vi "Format VI Information.vi"(0 "string in":string, 1 "output dir":path, 5 "file paths":path[](array[path]), 7 "image dir":path, 11 "error in":errorcluster) -> (4 "string out":string, 15 "error out":errorcluster)   [LabVIEW 2019, in "MD Generator.lvlib"]
uses:
  MD Generator.lvlib
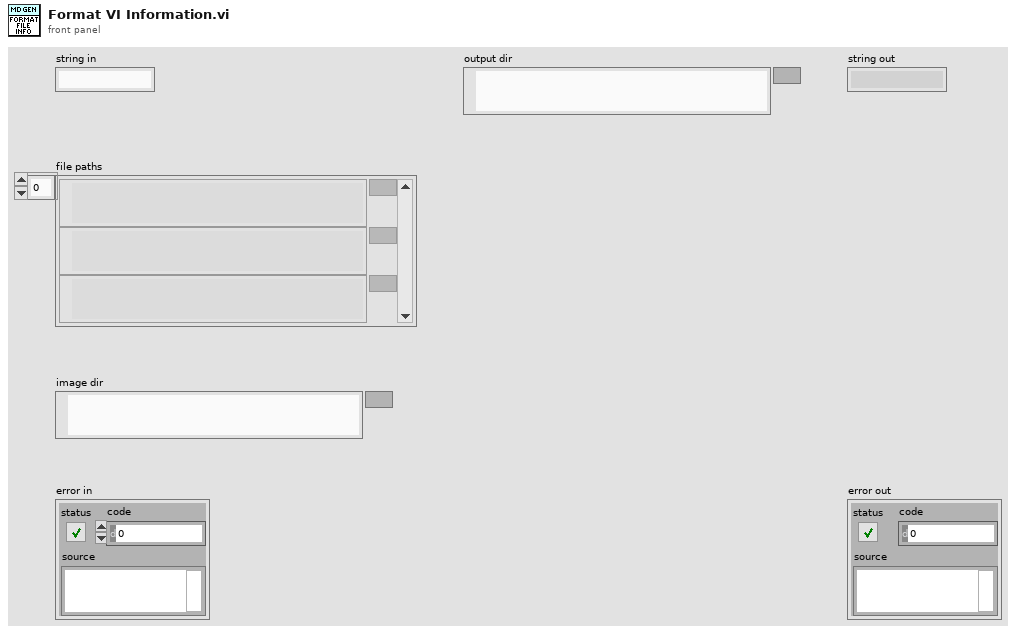
[diagram p1: front panel]
types:
  T1 = enum32{"Custom", "Standard", "Using Panel", "Using SubVI", "Complete"}
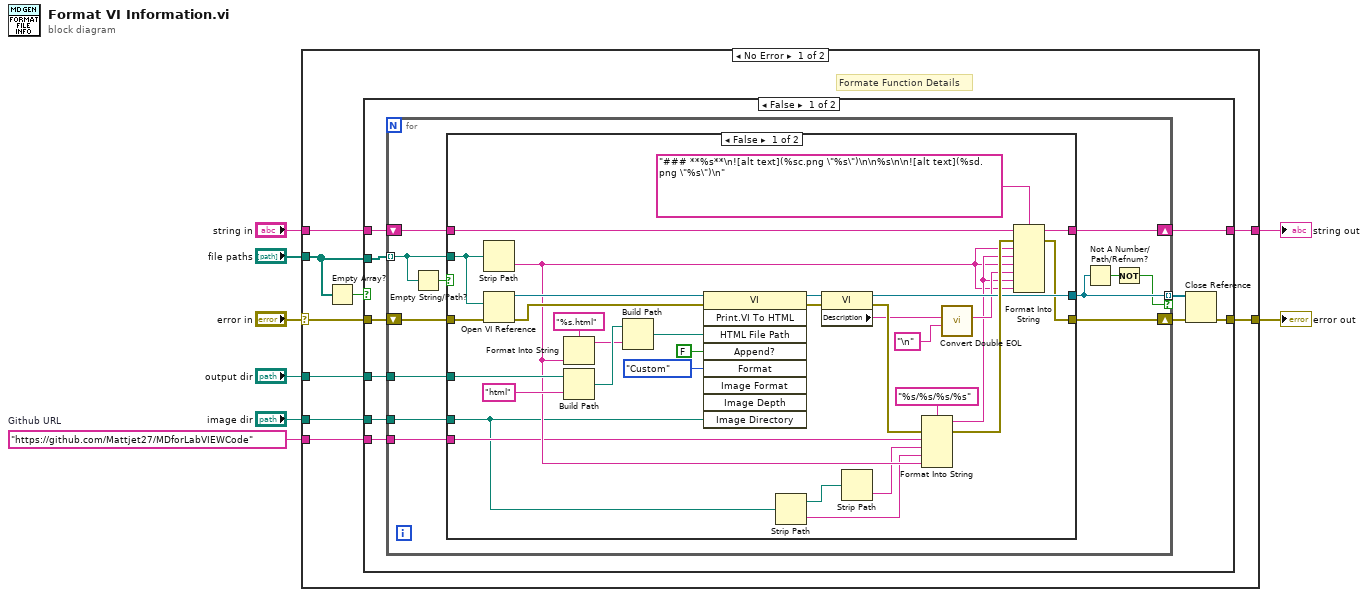
[diagram p0: block diagram]
diagram:
  w1 = "https://github.com/Mattjet27/MDforLabVIEWCode"  # Github URL
  n1 = case shown="No Error" "error in" {
    selector: "error in" -> [w16 w77]
    tunnel: [w17 w77] -> w8
    tunnel: "file paths" -> [w15 _]
    tunnel: "string in" -> [w14 w76]
    tunnel: [w12 w76] -> w4
    tunnel: "image dir" -> [w11 _]
    tunnel: "output dir" -> [w10 _]
    tunnel: w1 -> [w9 _]
    frame No Error {
      # "Formate Function Details"
      n2 = Empty Array?(array=w15) -> (empty?=w13:bool)
      n3 = case shown="False" w13 {
        tunnel: w14 -> [w27 w75]
        tunnel: [w26 w75] -> w12
        tunnel: w15 -> [w25 _]
        tunnel: [w22 w74] -> w17
        tunnel: w16 -> [w24 w74]
        tunnel: w11 -> [w20 _]
        tunnel: w10 -> [w19 _]
        tunnel: w9 -> [w18 _]
        frame False {
          n4 = for {
            shift-right: [w38] -> w26
            shift-left: w27 -> [w39]
            tunnel: w25 -> [w35] mode=indexing
            tunnel: [w32] -> w23 mode=indexing if=w31
            shift-right: [w36] -> w21
            shift-left: w24 -> [w37]
            tunnel: w20 -> [w30]
            tunnel: w19 -> [w29]
            tunnel: w18 -> [w28]
            n5 = Empty String/Path?(string/path=w35) -> (empty?=w34:bool)
            n6 = case shown="False" w34 {
              tunnel: w39 -> [w69 w72]
              tunnel: [w68 w72] -> w38
              tunnel: w35 -> [w65 _]
              tunnel: w37 -> [w64 w73]
              tunnel: [w63 _] -> w32
              tunnel: [w62 w73] -> w36
              tunnel: w30 -> [w43 _]
              tunnel: w29 -> [w49 _]
              tunnel: w28 -> [w44 _]
              frame False {
                n7 = Strip Path(path=w65) -> (name=w45:string)  [unwired: 1 out]
                n8 = Open VI Reference(vi path=w65, error in (no error)=w64) -> (vi reference=w58:refnum<vi>, error out=w66:errorcluster)  [unwired: 4 in]
                n9 = Format Into String(format string="%s.html", w45) -> (resulting string=w51:string)  [unwired: 2 in, 1 out]
                n10 = Build Path(base path=w49, name or relative path="html") -> (appended path=w53:path)
                n11 = Build Path(base path=w53, name or relative path=w51) -> (appended path=w52:path)
                n12 = invoke class="VI" method="Print.VI To HTML"(reference=w58, error in=w66, "HTML File Path"=w52, "Append?"=FALSE, "Format"=T1."Custom", "Image Directory"=w43) -> (reference out=w57:refnum<vi>, error out=w59:errorcluster)  [unwired: 3 in, 7 out]
                n13 = Strip Path(path=w43) -> (stripped path=w42:path, name=w40:string)
                n14 = property class="VI"(reference=w57, error in=w59) -> (reference out=w63:refnum<vi>, error out=w71:errorcluster, "Description"=w61:string)
                n15 = Strip Path(path=w42) -> (name=w41:string)  [unwired: 1 out]
                n16 = Format Into String(format string="%s/%s/%s/%s", error in=w71, w44, w41, w40, w45) -> (resulting string=w46:string, error out=w70:errorcluster)  [unwired: 1 in]
                n17 = call "Convert Double EOL.vi"("convert to"="\n", "string in"=w61) -> ("string out"=w47:string)  [unwired: 9 in]
                n18 = Format Into String(format string="### **%s**\n![alt text](%sc.png \"%s\")\n\n%s\n\n![alt text](%sd.png \"%s\")\n", initial string=w69, error in=w70, w45, w46, w45, w47, w46, w45) -> (resulting string=w68:string, error out=w62:errorcluster)
              }
              frame True {
              }
            }
            n19 = Not A Number/Path/Refnum?(number/path/refnum=w32) -> (NaN/Path/Refnum?=w33:bool)
            n20 = Not(x=w33) -> (.not. x?=w31:bool)
          }
          n21 = Close Reference(reference=w23, error in (no error)=w21) -> (error out=w22:errorcluster)
        }
        frame True {
        }
      }
    }
    frame Error {
    }
  }
  "error out" <- w8
  "string out" <- w4
